vi "chopperSetF.vi"(8 "error in (no error)":errorcluster, 10 "freq (Hz)":i16=1370, 11 "VISA Refnum in":refnum<visa-resource-name>) -> (0 "error out":errorcluster, 3 "VISA Refnum out":refnum<visa-resource-name>)   [LabVIEW 2011]
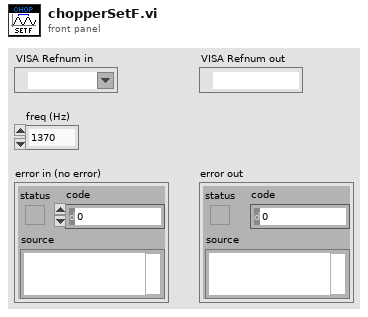
[diagram p1: front panel]
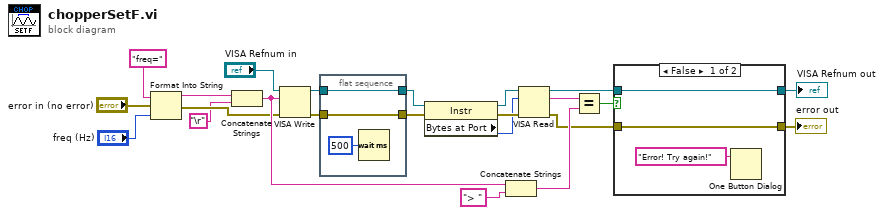
[diagram p0: block diagram]
diagram:
  n1 = Format Into String(initial string="freq=" ("write buffer"), error in="error in (no error)", "freq (Hz)") -> (resulting string=w16:string, error out=w19:errorcluster)  [unwired: 1 in]
  n2 = Concatenate Strings(w16, "\r") -> (w21:string)
  n3 = VISA Write(VISA resource name="VISA Refnum in", write buffer=w21, error in (no error)=w19) -> (VISA resource name out=w10:refnum<visa-resource-name>, error out=w13:errorcluster)  [unwired: 1 out]
  n4 = flat-sequence {
    tunnel: w10 -> [w26]
    tunnel: [w26] -> w11
    tunnel: [w25] -> w12
    tunnel: w13 -> [w25]
    frame #0 {
      n5 = Wait (ms)(milliseconds to wait=u32 500) -> ()  [unwired: 1 out]
    }
  }
  n6 = property class="Instr"(reference=w11, error in=w12) -> (reference out=w5:refnum<visa-resource-name>, error out=w4:errorcluster, "Bytes at Port"=w3:u32)
  n7 = Concatenate Strings(w21, "> " ("y")) -> (w22:string)
  n8 = VISA Read(VISA resource name=w5, byte count=w3, error in (no error)=w4) -> (VISA resource name out=w9:refnum<visa-resource-name>, read buffer=w6:string, error out=w8:errorcluster)  [unwired: 1 out]
  n9 = Equal?(x=w6, y=w22) -> (x = y?=w7:bool)
  n10 = case shown="False" w7 {
    tunnel: w8 -> [w28 w30]
    tunnel: w9 -> [w27 w31]
    tunnel: [w27 w31] -> w1
    tunnel: [w28 w30] -> w2
    frame False {
      n11 = One Button Dialog(message="Error! Try again!") -> ()  [unwired: 1 in, 1 out]
    }
    frame True {
    }
  }
  "VISA Refnum out" <- w1
  "error out" <- w2
